vi "Increase array size.vi"(1 "Array in":dbl[](array[numeric]) format="%.2f", 3 "Only if Array\nis not empty?":bool=TRUE, 4 "Size":i32) -> (15 "Array out":dbl[](array[numeric]) format="%.2f")   [LabVIEW 2020]
doc: "If size of Array in is smaller than Size, this VI increases the size of Array in to Size. If Array in is an empty array and Only if Array is not empty? is FALSE, VI builds an array of zeros with the size of Size."
panel:
  # "If size of Array in is smaller than Size, this VI increases \nthe size of Array in to Size.  If Array in is an empty array and \n\"Only if Array is not empty?\" is FALSE, VI builds an array of zeros with the size of Size."
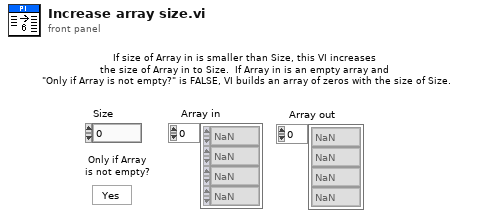
[diagram p1: front panel]
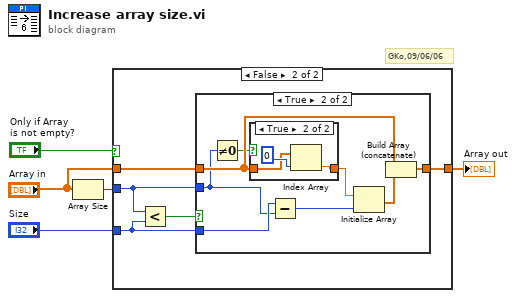
[diagram p0: block diagram]
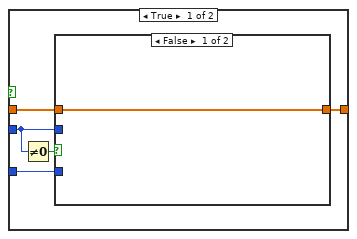
[diagram p2: hidden frame]
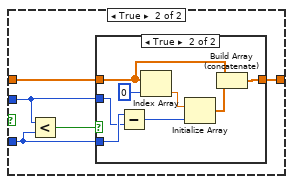
[diagram p3: hidden frame]
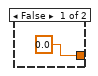
[diagram p6: hidden frame]
diagram:
  # "GKo,09/06/06"
  n1 = Array Size(array="Array in") -> (size(s)=w5:i32)
  n2 = case shown="False" "Only if Array\nis not empty?" {
    tunnel: w5 -> [w7 w26]
    tunnel: "Array in" -> [w9 w30]
    tunnel: [w8 w29] -> w1
    tunnel: "Size" -> [w6 w28]
    frame True {
      n3 = Not Equal To 0?(x=w7) -> (x != 0?=w10:bool)
      n4 = case shown="False" w10 {
        tunnel: w9 -> [w11 w13]
        tunnel: [w11 w12] -> w8
        tunnel: w7 -> [_ w15]
        tunnel: w6 -> [_ w14]
        frame False {
        }
        frame True {
          n5 = Less?(x=w15, y=w14) -> (x < y?=w16:bool)
          n6 = case shown="True" w16 {
            tunnel: w13 -> [w17 w22]
            tunnel: w15 -> [_ w18]
            tunnel: w14 -> [_ w19]
            tunnel: [w17 w20] -> w12
            frame False {
            }
            frame True {
              n7 = Subtract(x=w19, y=w18) -> (x-y=w25:i32)
              n8 = Index Array(array=w22, index=0) -> (element=w23:dbl)
              n9 = Initialize Array(w23, w25) -> (w21:dbl[])
              n10 = Build Array (concatenate)(w22, w21) -> (w20:dbl[])
            }
          }
        }
      }
    }
    frame False {
      n11 = Less?(x=w26, y=w28) -> (x < y?=w27:bool)
      n12 = case shown="True" w27 {
        tunnel: w30 -> [w31 w37]
        tunnel: w26 -> [_ w32]
        tunnel: w28 -> [_ w34]
        tunnel: [w31 w35] -> w29
        frame False {
        }
        frame True {
          n13 = Not Equal To 0?(x=w32) -> (x != 0?=w33:bool)
          n14 = case shown="True" w33 {
            tunnel: [0.0 w42] -> w38
            tunnel: w37 -> [_ w41]
            frame False {
            }
            frame True {
              n15 = Index Array(array=w41, index=0) -> (element=w42:dbl)
            }
          }
          n16 = Subtract(x=w34, y=w32) -> (x-y=w39:i32)
          n17 = Initialize Array(w38, w39) -> (w36:dbl[])
          n18 = Build Array (concatenate)(w37, w36) -> (w35:dbl[])
        }
      }
    }
  }
  "Array out" <- w1
